vi "TODO.vi"(8 "error in (no error)":errorcluster, 11 "Message":string) -> (0 "error out":errorcluster)   [LabVIEW 2013]
uses:
  030 - EVENTS/03 - ToMessageHandlerProcess/enumMessageCriticity.ctl
  090 - ERRORS/Ctrls/enumLogAndView.ctl
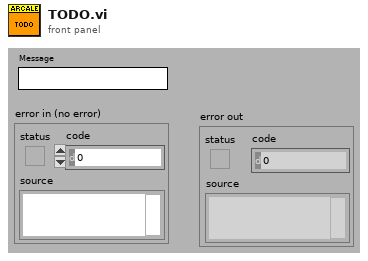
[diagram p1: front panel]
types:
  T1 = typedef "enumLogAndView.ctl" = enum16{"Log only", "Log and view"}
  T2 = typedef "enumMessageCriticity.ctl" = enum16{"No error", "Info", "Warning", "Error", "Fatal error"}
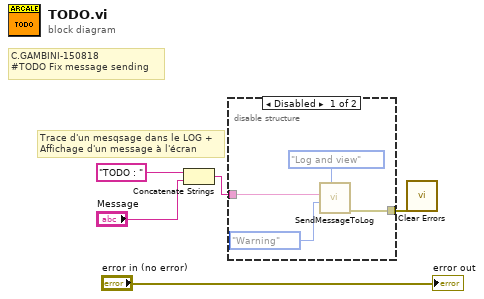
[diagram p0: block diagram]
diagram:
  # "C.GAMBINI-150818\n#TODO Fix message sending"
  # "Trace d'un mesqsage dans le LOG +\nAffichage d'un message à l'écran"
  n1 = Concatenate Strings("TODO : ", "Message") -> (w3:string)
  n2 = disable-structure shown="Disabled" {
    disable-tunnel: w3 -> [w9 _]
    disable-tunnel: [w7 _] -> w2
    frame Disabled {
      n3 = call "SendMessageToLog.vi"("Log and view ?"=enumLogAndView."Log and view", "Criticity"=enumMessageCriticity."Warning", "Message"=w9) -> ("error out"=w7:errorcluster)  [unwired: 7 in, 1 out]
    }
    frame Enabled {
    }
  }
  n4 = call <vilib>:"Clear Errors.vi"("error in (no error)"=w2) -> ()  [unwired: 6 in, 1 out]
  "error out" <- "error in (no error)"
